vi "Reset Unit.vi"(8 "error in (no error)":errorcluster, 11 "Ethernet in":refnum<class "ENET_BS1200.lvclass">) -> (0 "error out":errorcluster, 3 "Ethernet out":refnum<class "ENET_BS1200.lvclass">)   [LabVIEW 2021, in "BS120x Driver.lvlib" / "ENET_BS1200.lvclass"]
uses:
  ENET_BS1200.lvclass
  ENET_BS1200.lvclass/ENET_BS1200.ctl
  <vilib>/nisyscfg/Close (System).vi
  <vilib>/nisyscfg/nisyscfg.lvlib
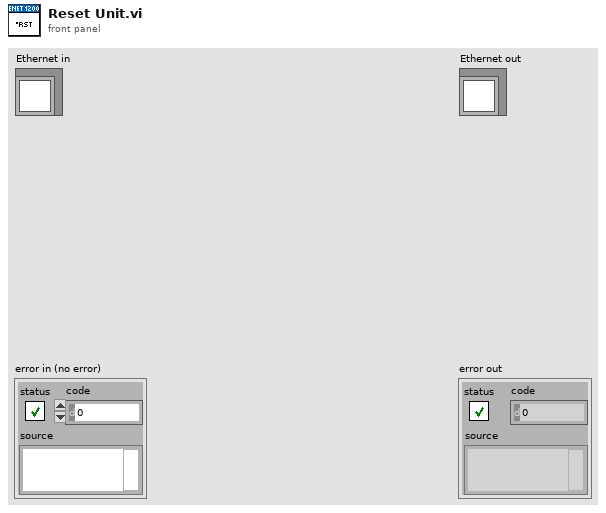
[diagram p1: front panel]
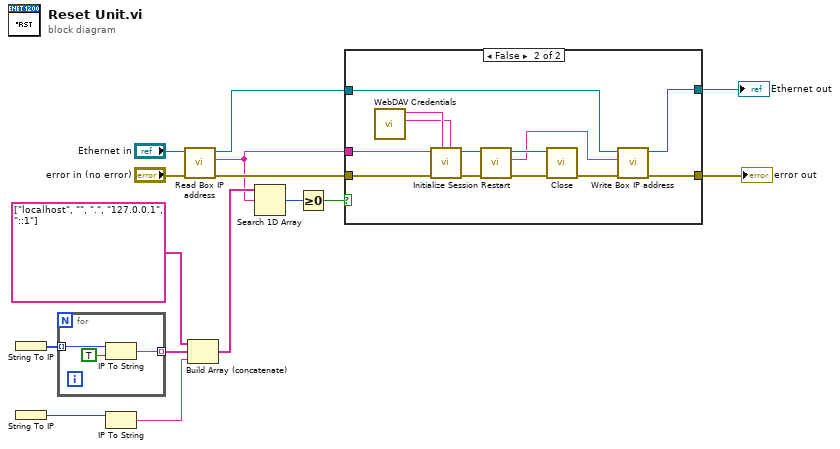
[diagram p0: block diagram]
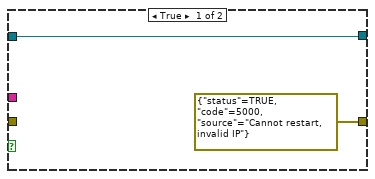
[diagram p2: hidden frame]
diagram:
  n1 = String To IP() -> (0:w9:u32[])  [unwired: 1 in]
  n2 = String To IP() -> (0:w6:u32)  [unwired: 1 in]
  n3 = for {
    tunnel: w9 -> [w18] mode=indexing
    tunnel: [w16] -> w8 mode=indexing
    n4 = IP To String(1:TRUE ("dot notation? (F)"), 2:w18) -> (0:w16:string)
  }
  n5 = IP To String(2:w6) -> (0:w5:string)  [unwired: 1 in]
  n6 = call-dynamic "Read Box IP address.vi"("error in (no error)"="error in (no error)", "ENET_BS120x in"="Ethernet in") -> ("error out"=w14:errorcluster, "Box IP address"=w1:string, "ENET_BS120x out"=w12:refnum<class "ENET_BS1200.lvclass">)  [unwired: 7 in]
  n7 = Build Array (concatenate)(string[] ["localhost", "", ".", "127.0.0.1", "::1"], w8, w5) -> (w4:string[])
  n8 = Search 1D Array(1D array=w4, element=w1) -> (index of element=w3:i32)  [unwired: 1 in]
  n9 = Greater Or Equal To 0?(x=w3) -> (x >= 0?=w2:bool)
  n10 = case shown="False" w2 {
    tunnel: w14 -> [_ w29]
    tunnel: w12 -> [w20 w27]
    tunnel: [w20 w26] -> w11
    tunnel: [errorcluster {"status"=TRUE, "code"=5000, "source"="Cannot restart, invalid IP"} ("error out") w25] -> w10
    tunnel: w1 -> [_ w21]
    frame True {
    }
    frame False {
      n11 = call "WebDAV Credentials.vi"() -> ("Password"=w22:string, "Username"=w23:string)  [unwired: 10 in]
      n12 = call <vilib>:"Initialize Session.vi"("Password"=w22, "User Name"=w23, "error in (no error)"=w29, "Target (localhost)"=w21) -> ("error out"=w33:errorcluster, "Session out"=w32:refnum<k21>)  [unwired: 6 in]
      n13 = call <vilib>:"Restart.vi"("error in (no error)"=w33, "Session in"=w32) -> ("error out"=w30:errorcluster, "New IP Address"=w24:string, "Session out"=w31:refnum<k21>)  [unwired: 7 in]
      n14 = call-poly <vilib>:"Close.vi"("error in (no error)"=w30, "Session in"=w31) -> ("error out"=w28:errorcluster)  [unwired: 9 in]
      n15 = call-dynamic "Write Box IP address.vi"("error in (no error)"=w28, "Box IP address"=w24, "ENET_BS120x in"=w27) -> ("error out"=w25:errorcluster, "ENET_BS120x out"=w26:refnum<class "ENET_BS1200.lvclass">)  [unwired: 7 in]
    }
  }
  "error out" <- w10
  "Ethernet out" <- w11
